vi "LDT Parse XML RA.vi"(8 "error in (no error)":errorcluster, 11 "XML RA":string="        <hours>12</hours>\n        <minutesTime>10</minutesTime>\n        <secondsTime>35.34</secondsTime>\n") -> (0 "error out":errorcluster, 2 "RA string":string, 3 "Position.RA":dbl)   [LabVIEW 2022 SP3, in "LDT Telescope.lvclass"]
uses:
  LDT Telescope.lvclass
  LDT Telescope.lvclass/LDT Telescope.ctl
  Telescope.lvclass
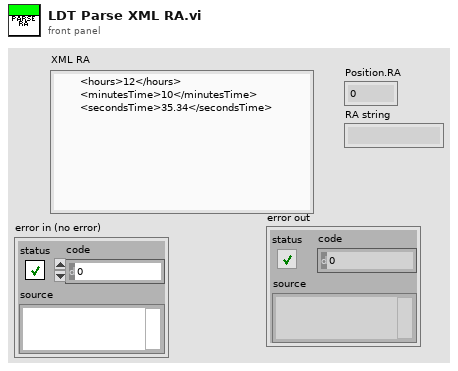
[diagram p1: front panel]
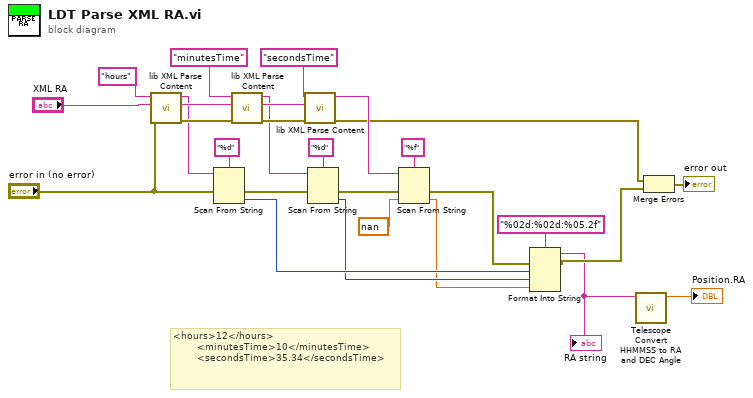
[diagram p0: block diagram]
diagram:
  # "<hours>12</hours>\n        <minutesTime>10</minutesTime>\n        <secondsTime>35.34</secondsTime>"
  n1 = call "lib XML Parse Content.vi"("error in (no error)"="error in (no error)", "XML Line"="XML RA", "XML Topic"="hours") -> ("error out"=w26:errorcluster, "XML Line dup"=w25:string, "Content"=w20:string)  [unwired: 6 in]
  n2 = Scan From String(format string="%d", input string=w20, error in="error in (no error)") -> (error out=w17:errorcluster, output 1=w9:i32)  [unwired: 2 in, 2 out]
  n3 = call "lib XML Parse Content.vi"("error in (no error)"=w26, "XML Line"=w25, "XML Topic"="minutesTime") -> ("error out"=w21:errorcluster, "XML Line dup"=w23:string, "Content"=w14:string)  [unwired: 6 in]
  n4 = call "lib XML Parse Content.vi"("error in (no error)"=w21, "XML Line"=w23, "XML Topic"="secondsTime") -> ("error out"=w4:errorcluster, "Content"=w13:string)  [unwired: 6 in, 1 out]
  n5 = Scan From String(format string="%d", input string=w14, error in=w17) -> (error out=w11:errorcluster, output 1=w8:i32)  [unwired: 2 in, 2 out]
  n6 = Scan From String(format string="%f", input string=w13, error in=w11, default 1=nan ("default value 1")) -> (error out=w6:errorcluster, output 1=w7:dbl)  [unwired: 1 in, 2 out]
  n7 = Format Into String(format string="%02d:%02d:%05.2f", error in=w6, w9, w8, w7) -> (resulting string=w2:string, error out=w5:errorcluster)  [unwired: 1 in]
  "RA string" <- w2
  n8 = call "Telescope Convert HHMMSS to RA and DEC Angle.vi"("RA String"=w2) -> ("RA"=→"Position.RA":dbl)  [unwired: 8 in, 2 out]
  n9 = Merge Errors(w4, w5) -> (→"error out":errorcluster)
